vi "Get configuration chain.vi"(8 "error in (no error)":errorcluster, 11 "StageSPIMBase in":refnum<class "StageSPIM.lvclass">) -> (0 "error out":errorcluster, 1 "class name":string[](array[string]), 2 "configuration chain":variant[](array[variant]), 3 "StageSPIMBase out":refnum<class "StageSPIM.lvclass">)   [LabVIEW 2012, in "StageSPIM.lvclass"]
doc: "Returns an array of variants containing the configuration clusters of each class in the inheritance chain (lowest child class first), together with an array of all class names in the inheritance chain.\n\nFor classes without configuration cluster, the configuration chain contains empty variants."
uses:
  StageSPIM.lvclass
  <vilib>/Distrio/Murmex/Murmex/Murmex.lvclass
  StageSPIM.lvclass/StageSPIM.ctl
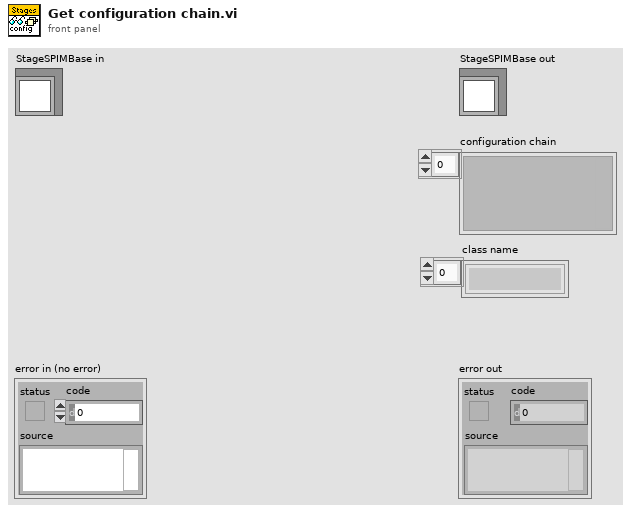
[diagram p1: front panel]
types:
  T1 = typedef "StageSPIM.lvclass/configuration_cluster.ctl" = cluster{"Port":T2, "Baudrate":T3, "Update frequency":dbl[unit], "S/N Master controller":string, "Interface":T4, "soft min limit":dbl[], "soft max limit":dbl[], "startup speedX":dbl[unit], "startup speedY":dbl[unit], "startup speedZ":dbl[unit], "startup speedFocus":dbl[unit]}
  T2 = typedef "StageSPIM.lvclass/port_control.ctl" = i32
  T3 = typedef "StageSPIM.lvclass/baud_rate_control.ctl" = u16
  T4 = typedef "StageSPIM.lvclass/connection_type.ctl" = enum16{"RS232", "RS232 DaisyChain", "USB", "USB_DaisyChain"}
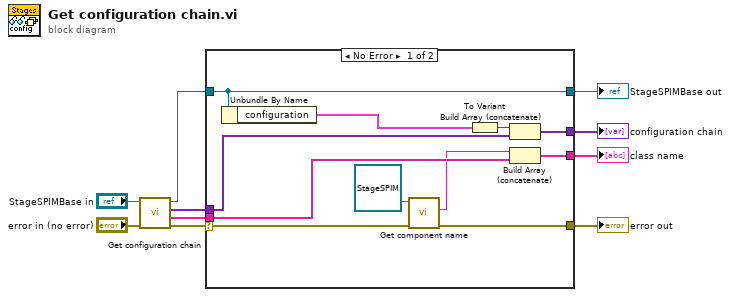
[diagram p0: block diagram]
diagram:
  n1 = call-parent "Get configuration chain.vi"("error in (no error)"="error in (no error)", "MurmexBase in"="StageSPIMBase in") -> ("error out"=w8:errorcluster, "class name"=w2:string[], "configuration chain"=w3:variant[], "MurmexBase out"=w6:refnum<class "StageSPIM.lvclass">)  [unwired: 6 in]
  n2 = case shown="No Error" w8 {
    selector: w8 -> [w21 w24]
    tunnel: [w20 w24] -> w7
    tunnel: w6 -> [w17 w25]
    tunnel: [w17 w25] -> w5
    tunnel: [w15 w22] -> w4
    tunnel: w3 -> [w14 w22]
    tunnel: w2 -> [w13 w23]
    tunnel: [w11 w23] -> w1
    frame No Error {
      n3 = Unbundle By Name(w17) -> ("configuration"=w16:T1)
      n4 = call <vilib>:"Get component name.vi"("error in (no error)"=w21, "Murmex in"=refnum<class "StageSPIM.lvclass"> refnum ("StageSPIM.lvclass")) -> ("error out"=w20:errorcluster, "component name"=w12:string)  [unwired: 7 in, 1 out]
      n5 = To Variant(anything=w16) -> (Variant=w18:variant)
      n6 = Build Array (concatenate)(w18, w14) -> (w15:variant[])
      n7 = Build Array (concatenate)(w12, w13) -> (w11:string[])
    }
    frame Error {
    }
  }
  "error out" <- w7
  "StageSPIMBase out" <- w5
  "configuration chain" <- w4
  "class name" <- w1
